vi "4.7.vi"() -> ()   [LabVIEW 2017]
panel:
  out "随机的数":i32
  out "猜测次数":i32
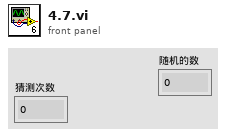
[diagram p1: front panel]
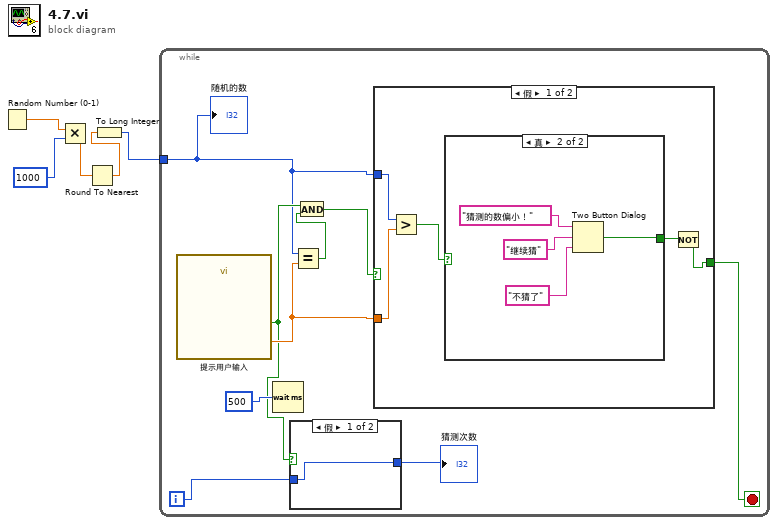
[diagram p0: block diagram]
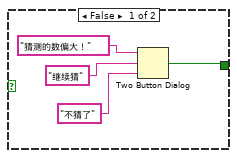
[diagram p3: hidden frame]
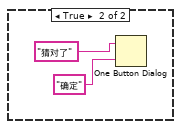
[diagram p4: hidden frame]
diagram:
  n1 = Random Number (0-1)() -> (number: 0 to 1=w5:dbl)
  n2 = Multiply(x=w5, y=1000) -> (x*y=w3:dbl)
  n3 = Round To Nearest(number=w3) -> (nearest integer value=w2:dbl)
  n4 = To Long Integer(number=w2) -> (32bit integer=w1:i32)
  n5 = while {
    tunnel: w1 -> [w6]
    i -> [w13]
    stop <- w8 stop-if-true
    n6 = call "提示用户输入"() -> ("请在1-1000猜"=w9:dbl, "确定"=w7:bool)  [unwired: 17 in, 1 out]
    n7 = Wait (ms)(milliseconds to wait=500) -> ()  [unwired: 1 out]
    n8 = case shown="假" w7 {
      tunnel: w13 -> [w15 _]
      tunnel: [w15 _] -> w12
      frame False {
      }
      frame True {
      }
    }
    "猜测次数" <- w12
    n9 = Equal?(x=w6, y=w9) -> (x = y?=w10:bool)
    n10 = And(x=w7, y=w10) -> (x .and. y?=w11:bool)
    n11 = case shown="假" w11 {
      tunnel: w6 -> [w20 _]
      tunnel: w9 -> [w19 _]
      tunnel: [w16 _] -> w8
      frame False {
        n12 = Greater?(x=w20, y=w19) -> (0:w18:bool)
        n13 = case shown="真" w18 {
          tunnel: [w21 w25] -> w17
          frame False {
            n14 = Two Button Dialog(message="猜测的数偏大！", 1:"不猜了", 2:"继续猜") -> (T button?=w21:bool)
          }
          frame True {
            n15 = Two Button Dialog(message="猜测的数偏小！", 1:"不猜了", 2:"继续猜") -> (T button?=w25:bool)
          }
        }
        n16 = Not(x=w17) -> (.not. x?=w16:bool)
      }
      frame True {
        n17 = One Button Dialog(message="猜对了", button name ("OK")="确定") -> ()  [unwired: 1 out]
      }
    }
    "随机的数" <- w6
  }
